vi "QI_CloseLib.vi"(2 "error in (no error)":errorcluster, 3 "path to dll":path) -> (0 "error out":errorcluster, 1 "CloseLib err":i32)   [LabVIEW 2014]
panel:
  in  "i":i32
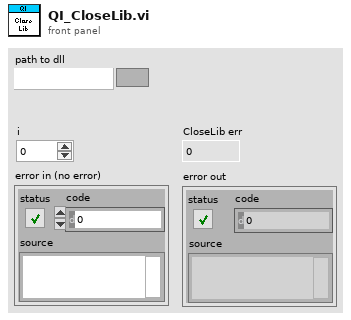
[diagram p1: front panel]
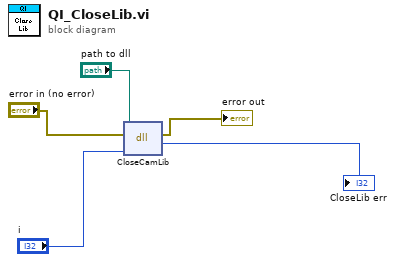
[diagram p0: block diagram]
diagram:
  n1 = dll-call lib="C:/Users/appli/Documents/Aline/octo-labview/QImaging/Release/QImaging.dll" fn="CloseCamLib"(path in="path to dll", error in="error in (no error)", "i"="i") -> (error out=→"error out":errorcluster, "return type"=→"CloseLib err":i32)  [unwired: 2 in, 1 out]
